vi "Get Rx Configuration.vi"(8 "error in":errorcluster, 11 "custom device":T1 format="%.0x") -> (0 "error out":errorcluster, 2 "configuration string out":string, 3 "custom device out":T1 format="%.0x")   [LabVIEW 2020, in "Ballard ARINC 429 Hardware Configuration.lvlib"]
uses:
  Ballard ARINC 429 Hardware Configuration.lvlib
  <vilib>/NI VeriStand/Custom Device API/Custom Device Item Ref.ctl
  Constants.vi
  Scripting/Ballard/Ballard ARINC 429 Scripting.lvlib
  Scripting/ARINC 429/ARINC 429 Scripting.lvlib
  <vilib>/NI VeriStand/Custom Device API/Custom Device API.lvlib
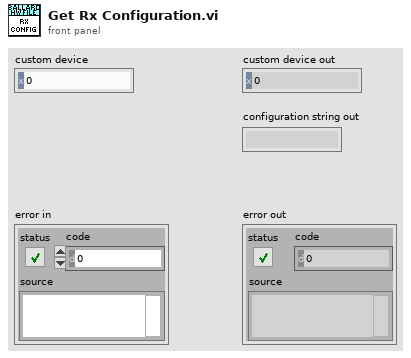
[diagram p1: front panel]
types:
  T1 = typedef "Custom Device API.lvlib/Custom Device Item Ref.ctl" = u64
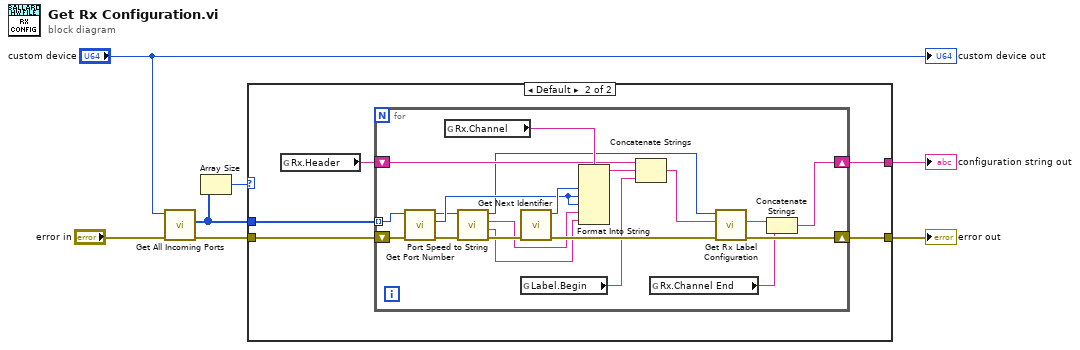
[diagram p0: block diagram]
diagram:
  n1 = call "Get All Incoming Ports.vi"("error in"="error in", "Ballard ARINC 429 custom device in"="custom device") -> ("error out"=w5:errorcluster, "incoming ports"=w2:T1[])  [unwired: 7 in, 1 out]
  n2 = Array Size(array=w2) -> (size(s)=w1:i32)
  n3 = case shown="Default" w1 {
    tunnel: w2 -> [_ w13]
    tunnel: w5 -> [w8 w12]
    tunnel: [_ w11] -> w4
    tunnel: [w8 w10] -> w3
    frame ..0 {
    }
    frame Default {
      n4 = global read "Constants.vi" "Rx.Header"() -> (w9:string)
      n5 = for {
        tunnel: w13 -> [w32] mode=indexing
        shift-right: [w24] -> w10
        shift-left: w12 -> [w33]
        shift-right: [w21] -> w11
        shift-left: w9 -> [w28]
        n6 = call "Get Port Number.vi"("error in"=w33, "port ref in"=w32) -> ("error out"=w19:errorcluster, "port number"=w29:u16, "port ref out"=w18:T1)  [unwired: 6 in, 1 out]
        n7 = global read "Constants.vi" "Rx.Channel"() -> (w31:string)
        n8 = call "Port Speed to String.vi"("error in"=w19, "port"=w18) -> ("error out"=w16:errorcluster, "speed string"=w14:string, "mode string"=w15:string, "port out"=w17:T1)  [unwired: 6 in]
        n9 = call "Get Next Identifier.vi"("error in"=w16) -> ("error out"=w25:errorcluster, "ID"=w30:u32)  [unwired: 9 in]
        n10 = global read "Constants.vi" "Label.Begin"() -> (w23:string)
        n11 = Format Into String(format string=w31, w30, w29, w29, w15, w14) -> (resulting string=w27:string)  [unwired: 2 in, 1 out]
        n12 = Concatenate Strings(w28, w27, w23) -> (w26:string)
        n13 = global read "Constants.vi" "Rx.Channel End"() -> (w20:string)
        n14 = call "Get Rx Label Configuration.vi"("error in"=w25, "configuration string"=w26, "port ref"=w17) -> ("error out"=w24:errorcluster, "configuration string out"=w22:string)  [unwired: 6 in, 1 out]
        n15 = Concatenate Strings(w22, w20) -> (w21:string)
      }
    }
  }
  "error out" <- w3
  "configuration string out" <- w4
  "custom device out" <- "custom device"
